vi "Select Robots By Confidence.vi"(11 "robots_blue":T1[](array[typedef]) {"height" format="%+4.3f"; "pixel_y" format="%+4.3f"; "pixel_x" format="%+4.3f"; "orientation" format="%+4.3f"; "y" format="%+4.3f"; "confidence" format="%4.3f"; "x" format="%+4.3f"}) -> (3 "Array":T1[](array[typedef]) {"height" format="%+4.3f"; "pixel_y" format="%+4.3f"; "pixel_x" format="%+4.3f"; "orientation" format="%+4.3f"; "y" format="%+4.3f"; "confidence" format="%4.3f"; "x" format="%+4.3f"})   [LabVIEW 2017]
uses:
  SSL Detection Robot.ctl
  <vilib>/Analysis/Matrix/Datatypes/RealMatrix.ctl
  <vilib>/Analysis/Matrix/NI_Matrix.lvlib
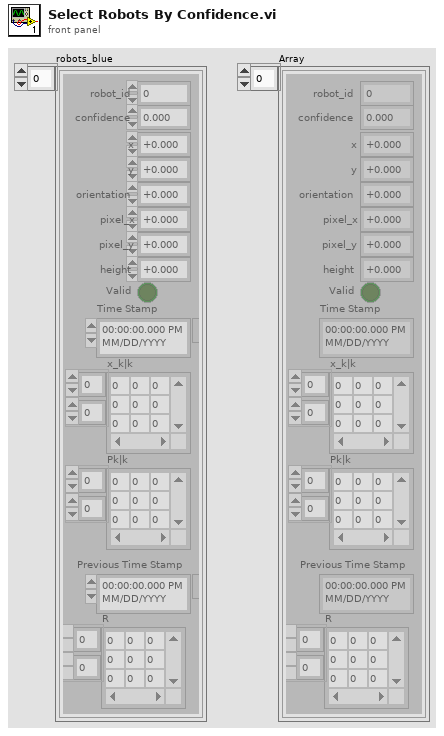
[diagram p1: front panel]
types:
  T1 = typedef "SSL Detection Robot.ctl" = cluster{"x":sgl, "robot_id":u32, "confidence":sgl, "y":sgl, "orientation":sgl, "pixel_x":sgl, "pixel_y":sgl, "height":sgl, "Valid":bool, "Time Stamp":timestamp, "x_k|k":T2, "Pk|k":T2, "Previous Time Stamp":timestamp, "R":T2}
  T2 = typedef "NI_Matrix.lvlib/RealMatrix.ctl" = dbl[][]
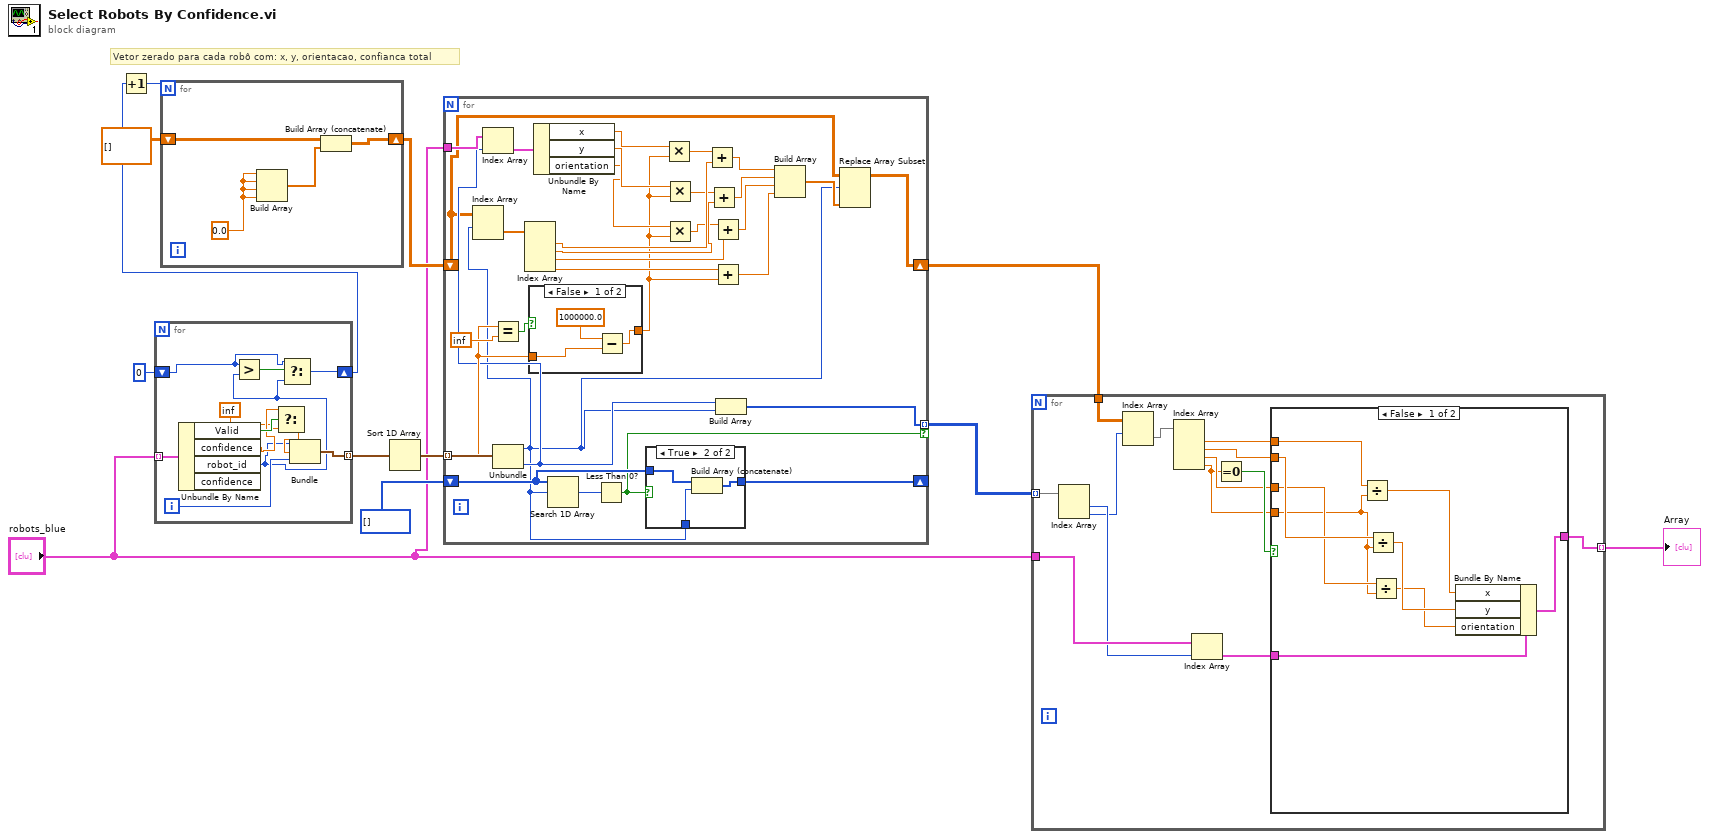
[diagram p0: block diagram]
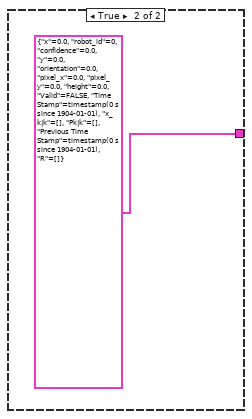
[diagram p2: hidden frame]
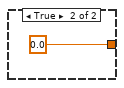
[diagram p3: hidden frame]
diagram:
  # "Vetor zerado para cada robô com: x, y, orientacao, confianca total"
  n1 = for {
    tunnel: "robots_blue" -> [w23] mode=indexing
    tunnel: [w22] -> w8 mode=indexing
    shift-right: [w13] -> w5
    shift-left: u32 0 ("robot_id") -> [w15]
    i -> [w21]
    n2 = Unbundle By Name(w23) -> ("Valid"=w20:bool, "confidence"=w19:sgl, "robot_id"=w14:u32)  [unwired: 1 out]
    n3 = Greater?(x=w15, y=w14) -> (0:w16:bool)
    n4 = Select(t=w19, s=w20, f=inf) -> (s? t:f=w18:dbl)
    n5 = Select(t=w15, s=w16, f=w14) -> (s? t:f=w13:u32)
    n6 = Bundle("robot_id"=w14, "confidence"=w18, w21) -> (w22:cluster{"robot_id":u32, "confidence":dbl, i32})  [unwired: 1 in]
  }
  n7 = Increment(x=w5) -> (x+1=w6:u32)
  n8 = for {
    N: w6 -> [_]
    shift-right: [w25] -> w3
    shift-left: dbl[][] [] -> [w26]
    w27 = 0.0 ("element")
    n9 = Build Array(w27, w27, w27, w27) -> (w24:dbl[])
    n10 = Build Array (concatenate)(w26, w24) -> (w25:dbl[][])
  }
  n11 = Sort 1D Array(array=w8) -> (sorted array=w9:cluster{"robot_id":u32, "confidence":dbl, i32}[])
  n12 = for {
    tunnel: w9 -> [w55] mode=indexing
    shift-right: [w57] -> _
    shift-left: i32[] [] -> [w58]
    tunnel: [w54] -> w11 mode=indexing if=w56
    shift-right: [w28] -> w1
    shift-left: w3 -> [w31]
    tunnel: "robots_blue" -> [w49]
    n13 = Unbundle(w55) -> ("robot_id"=w29:u32, "confidence"=w51:dbl, w47:i32)
    n14 = Index Array(array=w31, index (row)=w29) -> (element=w50:dbl[])  [unwired: 1 in]
    n15 = Index Array(array=w49, index=w47) -> (element=w48:T1)
    n16 = Equal?(x=w51, y=inf) -> (x = y?=w52:bool)
    n17 = Index Array(array=w50) -> (element #1=w42:dbl, element #2=w39:dbl, element #3=w36:dbl, element #4=w33:dbl)  [unwired: 4 in]
    n18 = case shown="False" w52 {
      tunnel: [w60 0.0 ("element")] -> w32
      tunnel: w51 -> [w61 _]
      frame False {
        n19 = Subtract(x=1000000.0, y=w61) -> (x-y=w60:dbl)
      }
      frame True {
      }
    }
    n20 = Unbundle By Name(w48) -> ("x"=w46:sgl, "y"=w45:sgl, "orientation"=w44:sgl)
    n21 = Search 1D Array(1D array=w58, element=w29) -> (index of element=w59:i32)  [unwired: 1 in]
    n22 = Less Than 0?(x=w59) -> (x < 0?=w56:bool)
    n23 = case shown="True" w56 {
      tunnel: w58 -> [w64 w67]
      tunnel: [w64 w66] -> w57
      tunnel: w29 -> [_ w65]
      frame False {
      }
      frame True {
        n24 = Build Array (concatenate)(w67, w65) -> (w66:u32[])
      }
    }
    n25 = Multiply(x=w46, y=w32) -> (x*y=w43:dbl)
    n26 = Multiply(x=w45, y=w32) -> (x*y=w40:dbl)
    n27 = Multiply(x=w44, y=w32) -> (x*y=w37:dbl)
    n28 = Add(x=w43, y=w42) -> (x+y=w41:dbl)
    n29 = Add(x=w40, y=w39) -> (x+y=w38:dbl)
    n30 = Add(x=w37, y=w36) -> (x+y=w35:dbl)
    n31 = Add(x=w33, y=w32) -> (x+y=w34:dbl)
    n32 = Build Array(w47, w29) -> (w54:u32[])
    n33 = Build Array(w41, w38, w35, w34) -> (w30:dbl[])
    n34 = Replace Array Subset(array=w31, new element=w30, index (row)=w29) -> (w28:dbl[][])  [unwired: 1 in]
  }
  n35 = for {
    tunnel: w11 -> [w79] mode=indexing
    tunnel: "robots_blue" -> [w80]
    tunnel: [w74] -> w12 mode=indexing
    tunnel: w1 -> [w77]
    n36 = Index Array(array=w79) -> (element #1=w78:u32, element #2=w76:u32)  [unwired: 2 in]
    n37 = Index Array(array=w77, index (row)=w76) -> (element=w75:dbl[])  [unwired: 1 in]
    n38 = Index Array(array=w75) -> (element #1=w72:dbl, element #2=w71:dbl, element #3=w70:dbl, element #4=w69:dbl)  [unwired: 4 in]
    n39 = Index Array(array=w80, index=w78) -> (element=w68:T1)
    n40 = Equal To 0?(x=w69) -> (x = 0?=w73:bool)
    n41 = case shown="False" w73 {
      tunnel: [w88 T1 {"x"=0.0, "robot_id"=0, "confidence"=0.0, "y"=0.0, "orientation"=0.0, "pixel_x"=0.0, "pixel_y"=0.0, "height"=0.0, "Valid"=FALSE, "Time Stamp"=timestamp(0 s since 1904-01-01), "x_k|k"=[], "Pk|k"=[], "Previous Time Stamp"=timestamp(0 s since 1904-01-01), "R"=[]} ("Detection Robot")] -> w74
      tunnel: w72 -> [w87 _]
      tunnel: w71 -> [w85 _]
      tunnel: w70 -> [w83 _]
      tunnel: w69 -> [w82 _]
      tunnel: w68 -> [w89 _]
      frame False {
        n42 = Divide(x=w87, y=w82) -> (x/y=w86:dbl)
        n43 = Divide(x=w85, y=w82) -> (x/y=w84:dbl)
        n44 = Divide(x=w83, y=w82) -> (x/y=w81:dbl)
        n45 = Bundle By Name(cluster=w89, "x"=w86, "y"=w84, "orientation"=w81) -> (w88:T1)
      }
      frame True {
      }
    }
  }
  "Array" <- w12
